vi "zsyrk - Symmetric Matrix Rank-k Update (CDB).vi"(4 "beta":cdb=1.0+0.0i, 6 "alpha":cdb=1.0+0.0i, 7 "operation A":T1 items=["Direct", "Conjugated & Transposed", "Transposed"], 8 "matrix C type":T2=3 items=["Lower Triangular"=2, "Upper Triangular"=3], 9 "C":T3, 11 "A":T3) -> (0 "error":i32, 3 "zsyrk":T3)   [LabVIEW 2017, in "NI_AALBLAS.lvlib"]
doc: "Calculates the rank-k update of the upper or lower triangular component of a symmetric matrix."
uses:
  <vilib>/Analysis/NI_AALBLAS.lvlib
  <vilib>/Analysis/Matrix/Datatypes/ComplexMatrix.ctl
  <vilib>/Analysis/BLAS.llb/LV_UpLo.ctl
  <vilib>/Analysis/BLAS.llb/LV_Transpose.ctl
  <vilib>/Analysis/BLAS.llb/Order.ctl
  <vilib>/Analysis/BLAS.llb/Fucntion.ctl
  <vilib>/Analysis/BLAS.llb/BLAS3 Utility(CDB).vi
  <vilib>/Analysis/Matrix/NI_Matrix.lvlib
panel:
  # "zsyrk=alpha*A*A'+beta*C / zsyrk=alpha*A'*A+beta*C"
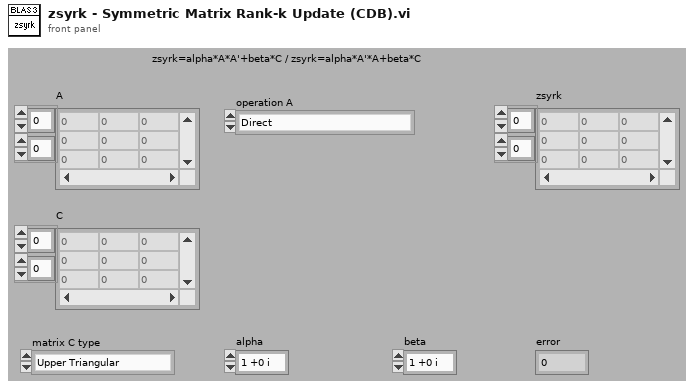
[diagram p1: front panel]
types:
  T1 = typedef "NI_AALBLAS.lvlib/LV_Transpose.ctl" = i32
  T2 = typedef "NI_AALBLAS.lvlib/LV_UpLo.ctl" = i32
  T3 = typedef "NI_Matrix.lvlib/ComplexMatrix.ctl" = cdb[][]
  T4 = typedef "NI_AALBLAS.lvlib/Fucntion.ctl" = u16
  T5 = typedef "NI_AALBLAS.lvlib/Order.ctl" = i32
  T6 = typedef "NI_AALBLAS.lvlib/Operation_Transpose.ctl" = i32
  T7 = typedef "NI_AALBLAS.lvlib/UpLo.ctl" = i32
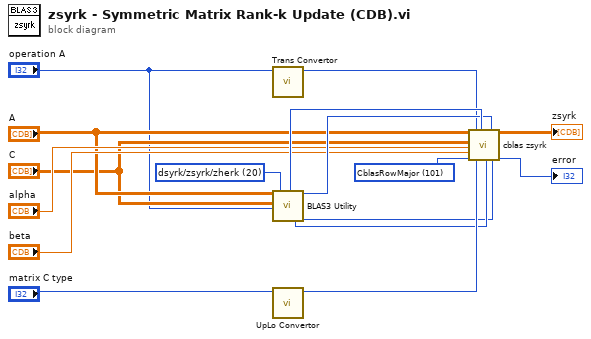
[diagram p0: block diagram]
diagram:
  w1 = T4 20 items=["ddot/zdotu/zdotc", "daxpy/zaxpy", "dnrm2/dznrm2", "dasum/dzasum", "dcopy/zcopy", "dswap/zswap", "drotm", "drot/zdrot", "idamax/izamax", "idamin/izamin", "dgemv/zgemv", "dsymv/zhemv", "dtrmv/ztrmv", "dsyr/zher", "dsyr2/zher2", "dger/zgeru/zgerc", "dtrsv/ztrsv", "dgemm/zgemm", "dsymm/zsymm/zhemm", "dtrmm/ztrmm", "dsyrk/zsyrk/zherk", "dsyr2k/zsyr2k/zher2k", "dtrsm/ztrsm"] ("function")
  w2 = T5 101 items=["CblasRowMajor"=101, "CblasColMajor"=102] ("order")
  n1 = call <vilib>:"Trans Convertor.vi"("operation"="operation A") -> ("trans"=w10:T6)  [unwired: 10 out]
  n2 = call-poly <vilib>:"BLAS3 Utility.vi"("A"="A", "C"="C", "operation A"="operation A", "function"=w1) -> ("lda"=w16:i32, "n"=w4:i32, "ldc"=w15:i32, "k"=w3:i32)  [unwired: 2 in, 10 out]
  n3 = call <vilib>:"UpLo Convertor.vi"("triangle matrix type"="matrix C type") -> ("uplo"=w11:T7)  [unwired: 10 out]
  n4 = call <vilib>:"cblas zsyrk.vi"("A"="A", "C"="C", "alpha"="alpha", "beta"="beta", "order"=w2, "transA"=w10, "uplo"=w11, "lda"=w16, "n"=w4, "ldc"=w15, "k"=w3) -> ("zsyrk"=→"zsyrk":T3, "error"=→"error":i32)  [unwired: 7 out]
